vi "[RT] Finite Acq wRearm.vi"() -> ()   [LabVIEW 2015]
doc: "When a finite acquisition terminates, the FPGA automatically rearms itself for another acquisition. You simply need to call rwfm_Start.vi to perform another finite acquisition."
uses:
  <vilib>/rvi/interface/nirviCloseFPGA/nirviCloseFPGA.xnode
  <vilib>/NI/cRIO Wfm/cRIO Wfm.lvlib
  <vilib>/NI/cRIO Wfm/AcqRead(Wfm).vi
  <vilib>/rvi/interface/nirviOpenFPGA/nirviOpenFPGA.xnode
  <vilib>/FPGAPlugInAG/cRIO-9074/niLvFpga_Open_cRIO-9074.vi
  <vilib>/rvi/interface/common/dynamic/niFpgaDynamicAddResources.vi
  <vilib>/FPGAPlugInAG/Dynamic/niLvFpga_Close_Dynamic.vi
  C:/Program Files (x86)/National Instruments/LabVIEW 2015/ProjectTemplates/Source/cRIOWfm/FPGA Bitfiles/DeltaSigMain_9074.lvbitx
  C:/Program Files (x86)/National Instruments/LabVIEW 2015/ProjectTemplates/Source/cRIOWfm/FPGA/[FPGA] DeltaSig Main.vi
  C:/Program Files (x86)/National Instruments/LabVIEW 2015/ProjectTemplates/Source/cRIOWfm/FPGA Bitfiles/SARAcqMain_9074.lvbitx
  C:/Program Files (x86)/National Instruments/LabVIEW 2015/ProjectTemplates/Source/cRIOWfm/FPGA/[FPGA] SAR Acq Main.vi
  <vilib>/NI/cRIO Wfm/ChannelConfig.ctl
panel:
  in  "Sample Rate":u32=51200
  in  "Channel Info":T1=[{"Channel Name"="Mod1/ai0", "Sensitivity mV_EU"=1000.0, "EU"="V", "dB Ref EU"=1.0}, {"Channel Name"="Mod1/ai1", "Sensitivity mV_EU"=1000.0, "EU"="V", "dB Ref EU"=1.0}, {"Channel Name"="Mod1/ai2", "Sensitivity mV_EU"=1000.0, "EU"="V", "dB Ref EU"=1.0}, {"Channel Name"="Mod1/ai3", "Sensitivity mV_EU"=1000.0, "EU"="V", "dB Ref EU"=1.0}] caption="Channel Name      Scale [mV/EU]        EU           dB Ref [EU]" {"dB Ref EU" format="%#.2p"; "Sensitivity mV_EU" format="%.2f"}
  in  "Samps per Chan":i32=25600 caption="Samples per Channel"
  in  "stop":bool
  out "Waveform Graph":waveform(sgl)[](graph)
  in  "Snapshot":bool
  # "Sampling Info"
  # "Channel Info"
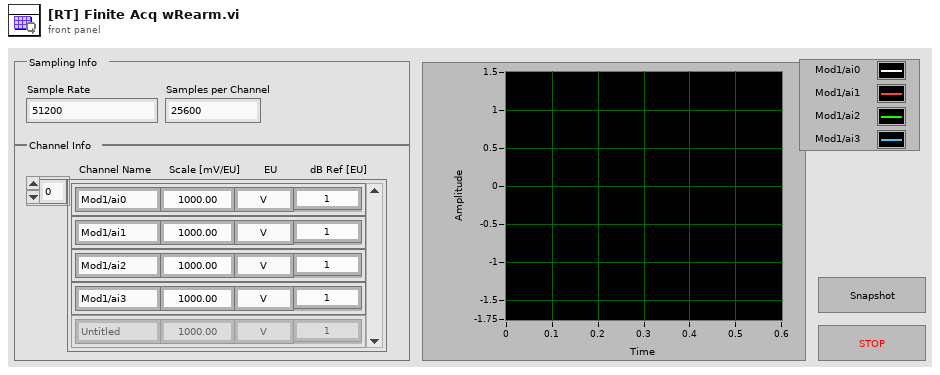
[diagram p1: front panel]
types:
  T1 = typedef "cRIO Wfm.lvlib/ChannelConfig.ctl" = cluster{"Channel Name":string, "Sensitivity mV_EU":dbl, "EU":string, "dB Ref EU":dbl}[]
  T2 = typedef "cRIO Wfm.lvlib/SamplingInfo.ctl" = cluster{"Number of Channels":i32, "Actual Samp Rate":dbl, "Chan Name Array":string[], "EU Chan Array":string[], "dB Ref Chan Array":dbl[]}
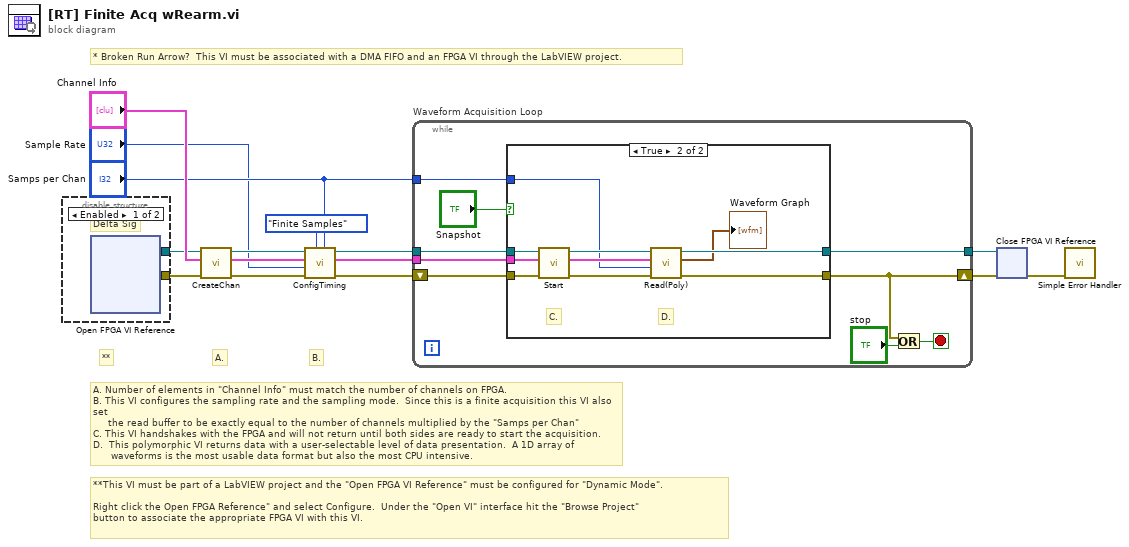
[diagram p0: block diagram]
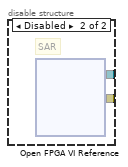
[diagram p2: hidden frame]
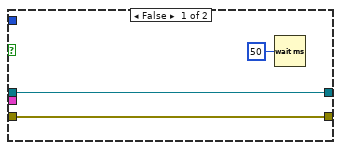
[diagram p3: hidden frame]
diagram:
  # "**This VI must be part of a LabVIEW project and the \"Open FPGA VI Reference\" must be configured for \"Dynamic Mode\".\n\nRight click the Open FPGA Reference\" and select Configure.  Under the \"Open VI\" interface hit the \"Browse Project\" \nbutton to associate the appropriate FPGA VI with this VI."
  # "* Broken Run Arrow?  This VI must be associated with a DMA FIFO and an FPGA VI through the LabVIEW project."
  # "A. Number of elements in \"Channel Info\" must match the number of channels on FPGA.\nB. This VI configures the sampling rate and the sampling mode.  Since this is a finite acquisition this VI also set  \n     the read buffer to be exactly equal to the number of channels multiplied by the \"Samps per Chan\"\nC. This VI handshakes with the FPGA and will not return until both sides are ready to start the acquisition.\nD.  This polymorphic VI returns data with a user-selectable level of data presentation.  A 1D array of     \n      waveforms is the most usable data format but also the most CPU intensive."
  # "**"
  # "B."
  # "A."
  n1 = disable-structure shown="Enabled" {
    disable-tunnel: [w17 w19] -> w2
    disable-tunnel: [w16 w18] -> w1
    frame Enabled {
      # "Delta Sig"
      n2 = xnode "Open FPGA VI Reference"() -> ("FPGA VI Reference Out"=w17:refnum<k20>, "error out"=w16:errorcluster)  [unwired: 2 in]
    }
    frame Disabled {
      # "SAR"
      n3 = xnode "Open FPGA VI Reference"() -> ("FPGA VI Reference Out"=w19:refnum<k20>, "error out"=w18:errorcluster)  [unwired: 2 in]
    }
  }
  n4 = call <vilib>:"CreateChan.vi"("error in"=w1, "Channel Info"="Channel Info", "Dynamic FPGA Ref"=w2) -> ("error out"=w7:errorcluster, "Sampling Info"=w6:T2, "Dynamic FPGA Ref Out"=w8:refnum<k20>)  [unwired: 1 in, 5 out]
  n5 = call <vilib>:"ConfigTiming.vi"("Samples per Channel"="Samps per Chan", "Sample Mode"=enum16{"Finite Samples", "Continuous Samples"}."Finite Samples", "error in"=w7, "Sample Rate"="Sample Rate", "Sampling Info In"=w6, "Dynamic FPGA Ref"=w8) -> ("error out"=w12:errorcluster, "Sampling Info Out"=w9:T2, "Dynamic FPGA Ref Out"=w13:refnum<k20>)  [unwired: 2 in, 1 out]
  n6 = while "Waveform Acquisition Loop" {
    tunnel: w13 -> [w27]
    tunnel: [w26] -> w11
    tunnel: w9 -> [w22]
    tunnel: "Samps per Chan" -> [w21]
    shift-right: [w20] -> w10
    shift-left: w12 -> [w28]
    stop <- w24 stop-if-true
    n7 = case shown="True" "Snapshot" {
      tunnel: w28 -> [w30 w41]
      tunnel: w27 -> [w31 w40]
      tunnel: [w31 w39] -> w26
      tunnel: [w30 w38] -> w20
      tunnel: w22 -> [_ w34]
      tunnel: w21 -> [_ w32]
      frame False {
        n8 = Wait (ms)(milliseconds to wait=u32 50) -> ()  [unwired: 1 out]
      }
      frame True {
        # "C."
        # "D."
        n9 = call <vilib>:"Start.vi"("error in"=w41, "Sampling Info In"=w34, "Dynamic FPGA Ref"=w40) -> ("error out"=w37:errorcluster, "Sampling Info Out"=w33:T2, "Dynamic FPGA Ref Out"=w36:refnum<k20>)  [unwired: 6 out]
        n10 = call-poly <vilib>:"Read(Poly).vi"("error in"=w37, "Samps Read per Chan"=w32, "Sampling Info"=w33, "Dynamic FPGA Ref"=w36) -> ("error out"=w38:errorcluster, "Wfm Data"=→"Waveform Graph":waveform(sgl)[], "Dynamic FPGA Ref Out"=w39:refnum<k20>)  [unwired: 2 in, 3 out]
      }
    }
    n11 = Or(x=w20, y="stop") -> (x .or. y?=w24:bool)
  }
  n12 = xnode "Close FPGA VI Reference"("FPGA VI Reference In"=w11, "error in"=w10) -> ("error out"=w14:errorcluster)
  n13 = call <vilib>:"Simple Error Handler.vi"("error in (no error)"=w14) -> ()  [unwired: 1 in, 8 out]
